vi "NIMS_DF_fir_nyquist(min,l,rf,ripple).vi"(7 "ripple":dbl=0.01 format="%#.6g", 9 "rolloff":dbl=0.01 format="%#.6g", 10 "l":i32=4, 11 "flag":enum16{"minorder"}(ring)) -> (0 "error":i32, 3 "b":dbl[](array[numeric]))   [LabVIEW 2017, in "NI_DigFilter_MathScript.lvlib"]
uses:
  <vilib>/addons/Digital Filter Design/NI_DigFilter_MathScript.lvlib
  <vilib>/addons/Digital Filter Design/NI_DigFilterLicensed.lvlib
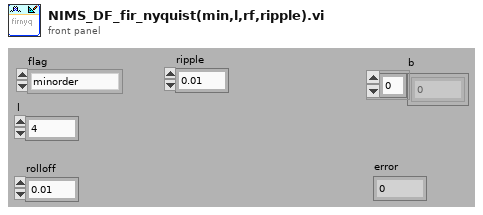
[diagram p1: front panel]
types:
  T1 = typedef "NI_DigFilterLicensed.lvlib/DFD Multirate Filter Obj.ctl" = cluster{"mMRate_Structure":enum16{"CIC", "FIR", "IIR", "Lattice"}, "mMRate_Mode":T2, "mMRate_Factor":i32, "mMRate_FIRParams":cluster{"mMRate_FIR_H":dbl[], "mMRate_FIR_IsNyquist?":bool, "mMRate_FIR_IsSymmetric?":bool}, "mMRate_CICParams":cluster{"mMRate_CIC_#Stage":i32, "mMRate_CIC_Lag":i32, "mMRate_CIC_Type":enum16{"Lowpass", "Highpass"}}, "mMRate_Order":i32, "mMRate_Version":string, "mMRate_Comments":string, "mMRate_RationalFactor":cluster{"mMRate_L":i32, "mMRate_M":i32}, "mMRate_Fs":dbl, "mMRate_Quantized?":bool, "mMRate_QFilterGain":dbl, "mMRate_CoefWl":i16, "mMRate_Scaling":cluster{"mMRate_ScaleByPowerOf2?":bool, "mMRate_ScaleType":T3}, "mMRate_InputWl":i16, "mMRate_OutputWl":i16, "mMRate_OutputMode":T4, "mMRate_MultMode":T5, "mMRate_BitPruning":bool, "mMRate_GainWl":i16, "mMRate_OutputFwl":i16, "mMRate_SumIwl":i16, "mMRate_InputIwl ":i16, "mMRate_SumWl":i16, "mMRate_CoefIwl":i16}
  T2 = typedef "NI_DigFilterLicensed.lvlib/DFD Multirate Mode.ctl" = i16
  T3 = typedef "NI_DigFilterLicensed.lvlib/DFD Coef Norm Type.ctl" = enum16{"No Norm", "Time Domain 1-Norm", "Time Domain 2-Norm", "Time Domain Inf-Norm"}
  T4 = typedef "NI_DigFilterLicensed.lvlib/DFD Round-off Mode.ctl" = enum16{"Nearest", "Truncation"}
  T5 = typedef "NI_DigFilterLicensed.lvlib/DFD FXP MRate Multiply Mode.ctl" = enum16{"Truncated", "Full"}
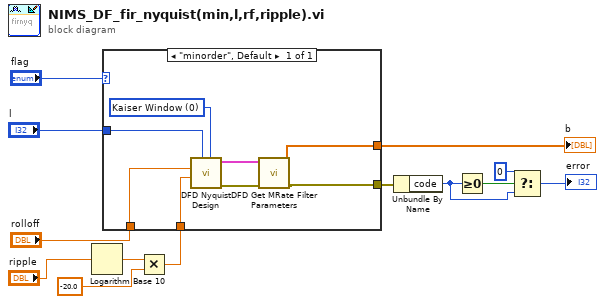
[diagram p0: block diagram]
diagram:
  n1 = Logarithm Base 10(1:"ripple") -> (0:w8:dbl)
  n2 = Multiply(x=w8, y=-20.0) -> (x*y=w6:dbl)
  n3 = case shown="\"minorder\", Default" "flag" {
    tunnel: "l" -> [w21]
    tunnel: "rolloff" -> [w20]
    tunnel: [w18] -> w2
    tunnel: [w16] -> w11
    tunnel: w6 -> [w14]
    frame "minorder", Default {
      w15 = u16 0 items=["Kaiser Window", "Dolph-Chebyshev Window", "Equi-Ripple", "Positive Equi-Ripple"] ("method")
      n4 = call <vilib>:"DFD Nyquist Design.vi"("method"=w15, "factor"=w21, "stopband attenuation [dB]"=w14, "roll off"=w20) -> ("error out"=w19:errorcluster, "multirate filter out"=w17:T1)  [unwired: 4 in, 2 out]
      n5 = call <vilib>:"DFD Get MRate Filter Parameters.vi"("error in (no error)"=w19, "multirate filter in"=w17) -> ("error out"=w18:errorcluster, "h(n)"=w16:dbl[])  [unwired: 1 in, 7 out]
    }
  }
  "b" <- w11
  n6 = Unbundle By Name(w2) -> ("code"=w4:i32)
  n7 = Greater Or Equal To 0?(x=w4) -> (x >= 0?=w5:bool)
  n8 = Select(t=0 ("error"), s=w5, f=w4) -> (s? t:f=→"error":i32)
